vi "Get conversion component.vi"(8 "error in (no error)":errorcluster, 11 "ImageStack in":refnum<class "Invivo_ImageStack.lvclass">) -> (0 "error out":errorcluster, 2 "Conversion component name":string, 3 "ImageStack out":refnum<class "Invivo_ImageStack.lvclass">)   [LabVIEW 2012, in "Invivo_ImageStack.lvclass"]
uses:
  Invivo_ImageStack.lvclass
  Invivo_ImageStack.lvclass/Invivo_ImageStack.ctl
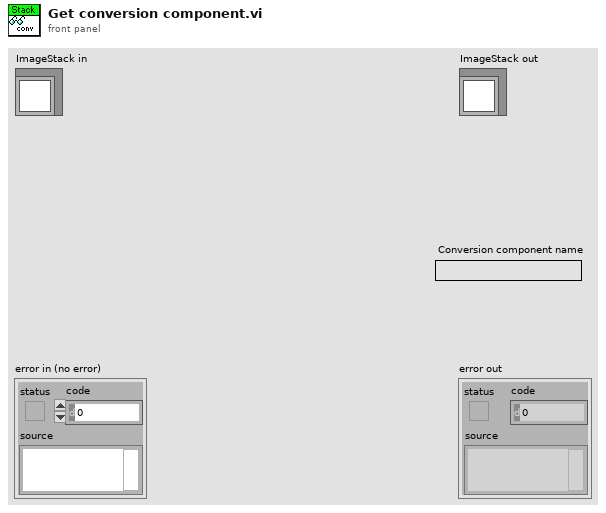
[diagram p1: front panel]
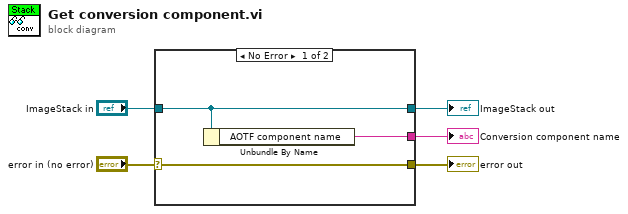
[diagram p0: block diagram]
diagram:
  n1 = case shown="No Error" "error in (no error)" {
    selector: "error in (no error)" -> [w8 w10]
    tunnel: [w8 w10] -> w4
    tunnel: [w7 w9] -> w2
    tunnel: "ImageStack in" -> [w7 w9]
    tunnel: [w6 _] -> w1
    frame No Error {
      n2 = Unbundle By Name(w7) -> ("AOTF component name"=w6:string)
    }
    frame Error {
    }
  }
  "error out" <- w4
  "ImageStack out" <- w2
  "Conversion component name" <- w1
